vi "Mod_OFDM_Continous_Phase_Complex_Symbols.vi"(0 "Complex Symbols w/ Cyclic prefix":cdb[](array[numeric]), 2 "Phase Continous":bool=TRUE, 7 "Pulse Shaping":T1={"System Filter"={"TX Filter"=enum."Root Raised Cos", "Alpha"=0.5, "filter length"=8}, "Modulation system parameters"={"samples per symbol (16)"=16}, "symbol rate (Hz)"=1.0} {"symbol rate (Hz)" min=1.0 step=1.0 format="%.2p"; "Modulation system parameters"."samples per symbol (16)" step=2; "System Filter"."Alpha" min=0.0 max=1.0 step=0.05 format="%.2f"}, 11 "error in (no error)":errorcluster) -> (3 "Size of Complex Symbols":i32, 4 "Complex Symbols w/ Cyclic prefix":cdb[](array[numeric]), 15 "error out":errorcluster)   [LabVIEW 2010]
uses:
  Controls(Type_DEf)/Configure Pulse Shaping.ctl
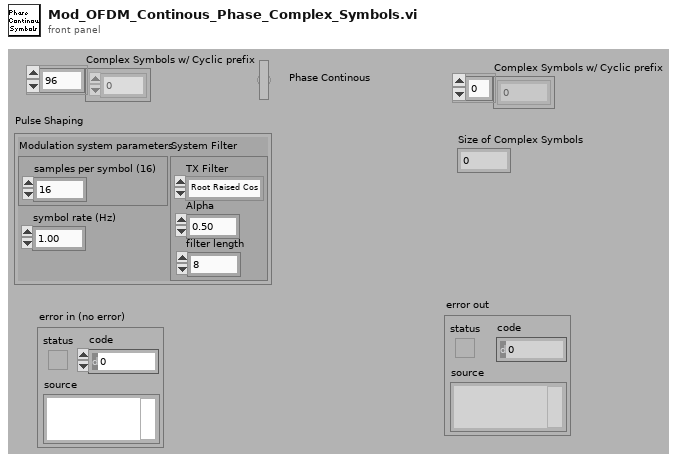
[diagram p1: front panel]
types:
  T1 = typedef "Configure Pulse Shaping.ctl" = cluster{"System Filter":cluster{"TX Filter":enum16{"none", "Raised Cosine", "Root Raised Cos"}, "Alpha":dbl, "filter length":i32}, "Modulation system parameters":cluster{"samples per symbol (16)":u32}, "symbol rate (Hz)":dbl}
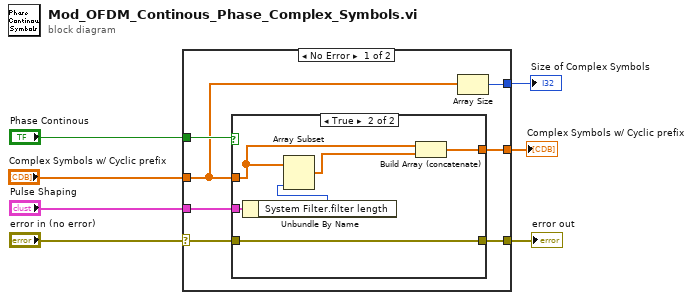
[diagram p0: block diagram]
diagram:
  n1 = case shown="No Error" "error in (no error)" {
    selector: "error in (no error)" -> [w11 w23]
    tunnel: [w10 w23] -> w6
    tunnel: "Pulse Shaping" -> [w13 _]
    tunnel: "Complex Symbols w/ Cyclic prefix" -> [w9 _]
    tunnel: "Phase Continous" -> [w14 _]
    tunnel: [w12 _] -> w2
    tunnel: [w8 _] -> w1
    frame No Error {
      n2 = case shown="True" w14 {
        tunnel: w9 -> [w15 w19]
        tunnel: w13 -> [_ w22]
        tunnel: [w15 w21] -> w12
        tunnel: w11 -> [w16 w20]
        tunnel: [w16 w20] -> w10
        frame False {
        }
        frame True {
          n3 = Unbundle By Name(w22) -> ("System Filter.filter length"=w17:i32)
          n4 = Array Subset(array=w19, length=w17) -> (w18:cdb[])  [unwired: 1 in]
          n5 = Build Array (concatenate)(w19, w18) -> (w21:cdb[])
        }
      }
      n6 = Array Size(array=w9) -> (size(s)=w8:i32)
    }
    frame Error {
    }
  }
  "error out" <- w6
  "Complex Symbols w/ Cyclic prefix" <- w2
  "Size of Complex Symbols" <- w1
